vi "видео 1.vi"() -> ()   [LabVIEW 2011]
uses:
  <vilib>/userDefined/High Color/IMAQdx.ctl
  <vilib>/vision/driver/NI_Vision_Acquisition_Software.lvlib
  <vilib>/vision/NI_Vision_Development_Module.lvlib
panel:
  out "Waveform Chart":i16(graph)
  in  "Numeric":i16
  in  "milliseconds to wait":u32
  in  "Truncation Frequency %":sgl=10.0 format="%.2f"
  in  "фильтр":bool
  in  "обработка":bool
  in  "Color Box 2":u32(colorbox)
  in  "Range":cluster{"Lower value":sgl, "Upper value":sgl}={"Lower value"=128.0, "Upper value"=255.0} {"Upper value" format="%.2f"; "Lower value" format="%.2f"}
  in  "out":i32
  out "Out (dis)":string
  in  "max out":i16
  out "max Out (dis)":string
  out "Boolean":bool
  in  "vc0":i16
  in  "Регулятор":bool
  in  "PV_зазор":i32
  out "PV  зазор (мм)":string
  out "SP  зазор (мм)":string
  in  "SP_зазор":i16
  in  "stop 3":bool
  in  "stop 2":bool
  out "16bit integer":i16
  out "x*y":dbl
  out "x/y":dbl
  out "Distance деталь":sgl format="%.2f"
  out "Coordinate System деталь (duplicate)":T1 {"Measurement System"."Axis Reference" items=["Direct", "Indirect"]; "Measurement System"."Angle (deg)" format="%.2f"; "Measurement System"."Origin"."Y" format="%.2f"; "Measurement System"."Origin"."X" format="%.2f"; "Reference System"."Axis Reference" items=["Direct", "Indirect"]; "Reference System"."Angle (deg)" format="%.2f"; "Reference System"."Origin"."Y" format="%.2f"; "Reference System"."Origin"."X" format="%.2f"}
  out "Edge Coordinates деталь":cluster{"X":sgl, "Y":sgl}[](array[cluster]) {"Y" format="%.2f"; "X" format="%.2f"}
  in  "Settingsдеталь":T2={"Contrast"=40, "Filter width"=4, "Steepness"=2, "Subsampling Ratio"=5, "Show Search Area"=FALSE, "Show Search Lines"=FALSE, "Show Edges Found"=FALSE, "Show Result"=TRUE}
  in  "Coordinate System деталь":T1 {"Measurement System"."Axis Reference" items=["Direct", "Indirect"]; "Measurement System"."Angle (deg)" format="%.2f"; "Measurement System"."Origin"."Y" format="%.2f"; "Measurement System"."Origin"."X" format="%.2f"; "Reference System"."Axis Reference" items=["Direct", "Indirect"]; "Reference System"."Angle (deg)" format="%.2f"; "Reference System"."Origin"."Y" format="%.2f"; "Reference System"."Origin"."X" format="%.2f"}
  in  "Rectangle деталь":T3 {"Rotation" format="%.2f"; "Left" scale=0.0..1024.0; "Right" scale=0.0..1024.0}
  in  "Color Plane":i32(ring)=1 items=["Red", "Green", "Blue", "Hue", "Saturation", "Luminance", "Value", "Intensity"]
  out "Edge Coordinates зазор":cluster{"X":sgl, "Y":sgl}[](array[cluster]) {"Y" format="%.2f"; "X" format="%.2f"}
  out "Distance зазор":sgl format="%.2f"
  out "Coordinate System зазор (duplicate)":T1 {"Measurement System"."Axis Reference" items=["Direct", "Indirect"]; "Measurement System"."Angle (deg)" format="%.2f"; "Measurement System"."Origin"."Y" format="%.2f"; "Measurement System"."Origin"."X" format="%.2f"; "Reference System"."Axis Reference" items=["Direct", "Indirect"]; "Reference System"."Angle (deg)" format="%.2f"; "Reference System"."Origin"."Y" format="%.2f"; "Reference System"."Origin"."X" format="%.2f"}
  in  "Coordinate System зазор":T1 {"Measurement System"."Axis Reference" items=["Direct", "Indirect"]; "Measurement System"."Angle (deg)" format="%.2f"; "Measurement System"."Origin"."Y" format="%.2f"; "Measurement System"."Origin"."X" format="%.2f"; "Reference System"."Axis Reference" items=["Direct", "Indirect"]; "Reference System"."Angle (deg)" format="%.2f"; "Reference System"."Origin"."Y" format="%.2f"; "Reference System"."Origin"."X" format="%.2f"}
  in  "Settings зазор":T2={"Contrast"=40, "Filter width"=4, "Steepness"=2, "Subsampling Ratio"=5, "Show Search Area"=FALSE, "Show Search Lines"=FALSE, "Show Edges Found"=FALSE, "Show Result"=TRUE}
  in  "Rectangle зазор":T3 {"Rotation" format="%.2f"; "Left" scale=0.0..1024.0; "Right" scale=0.0..1024.0}
  in  "Color Box":u32(colorbox)
  out "Image":T4(plugin-control)
  in  "stop":bool
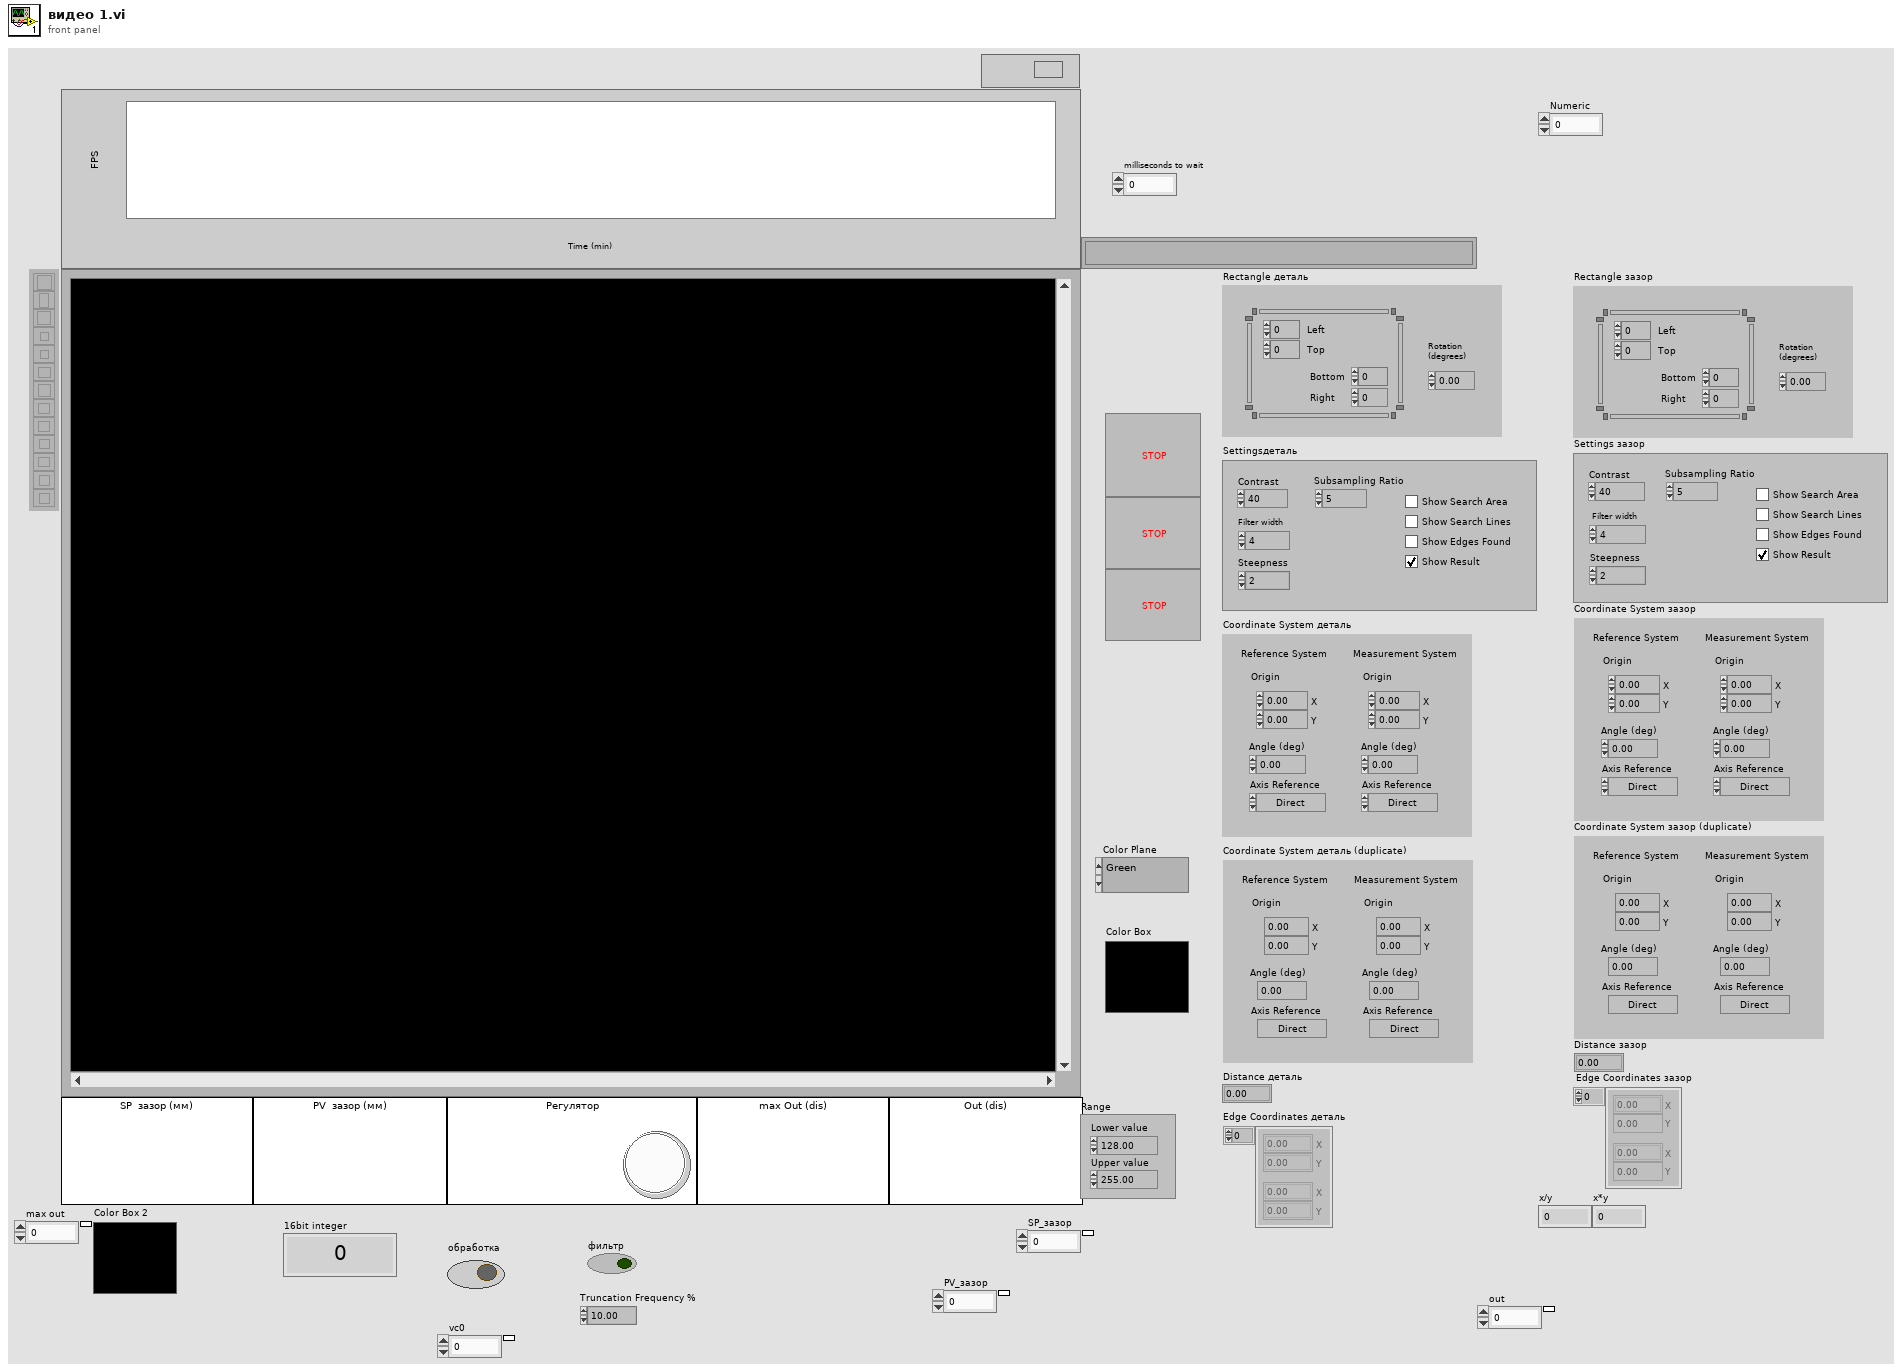
[diagram p1: front panel]
types:
  T1 = typedef "IMAQ Coordinate System" = cluster{"Reference System":cluster{"Origin":cluster{"X":sgl, "Y":sgl}, "Angle (deg)":sgl, "Axis Reference":u32}, "Measurement System":cluster{"Origin":cluster{"X":sgl, "Y":sgl}, "Angle (deg)":sgl, "Axis Reference":u32}}
  T2 = cluster{"Contrast":i32, "Filter width":i32, "Steepness":i32, "Subsampling Ratio":u32, "Show Search Area":bool, "Show Search Lines":bool, "Show Edges Found":bool, "Show Result":bool}
  T3 = typedef "IMAQ Rectangle" = cluster{"Left":i32, "Top":i32, "Right":i32, "Bottom":i32, "Rotation":dbl}
  T4 = typedef "IMAQ Image.ctl" = refnum<image>
  T5 = typedef "Image Type" = u32
  T6 = typedef "IMAQdx.ctl" = refnum<k21>
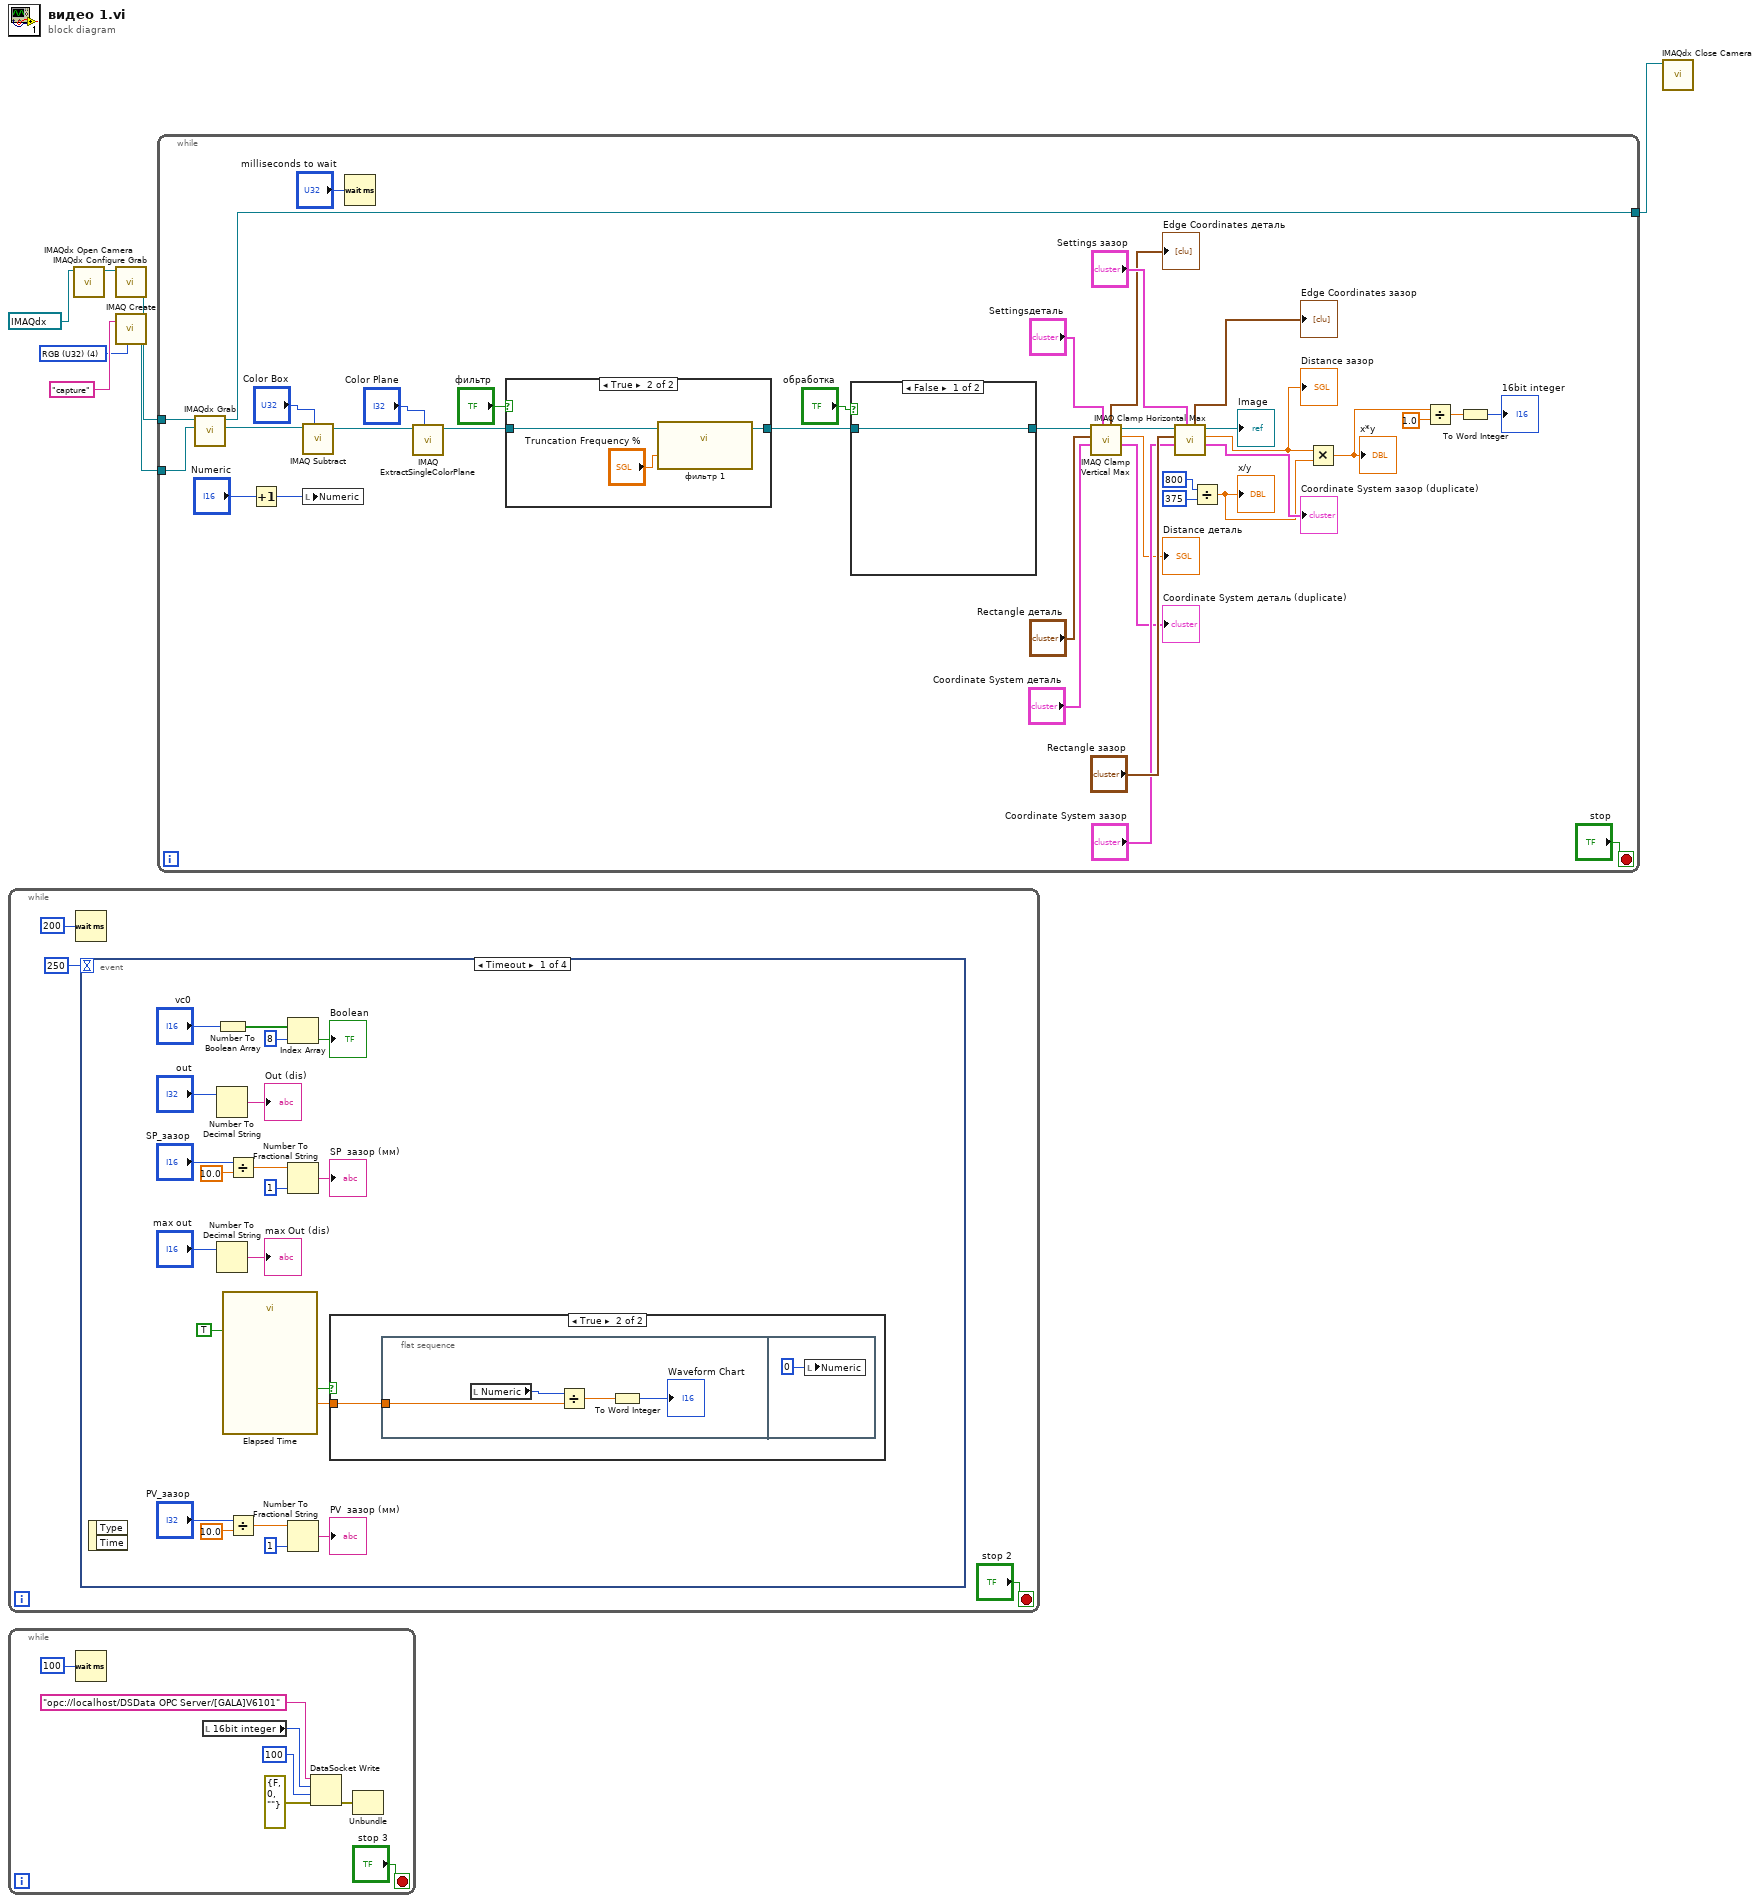
[diagram p0: block diagram]
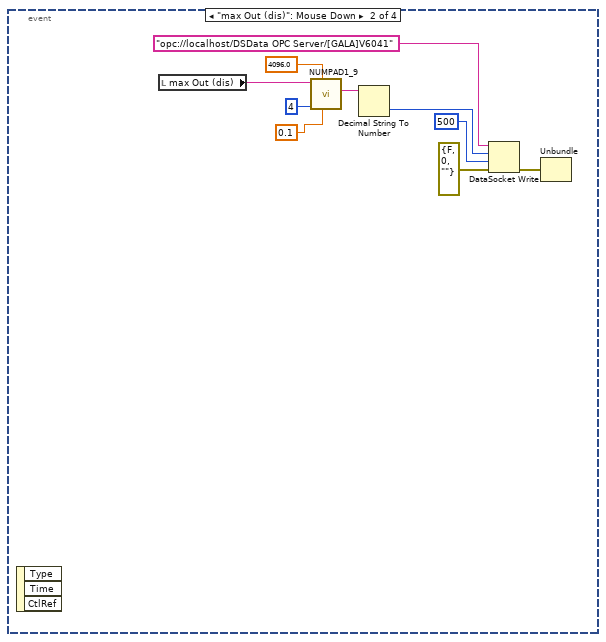
[diagram p3: hidden frame]
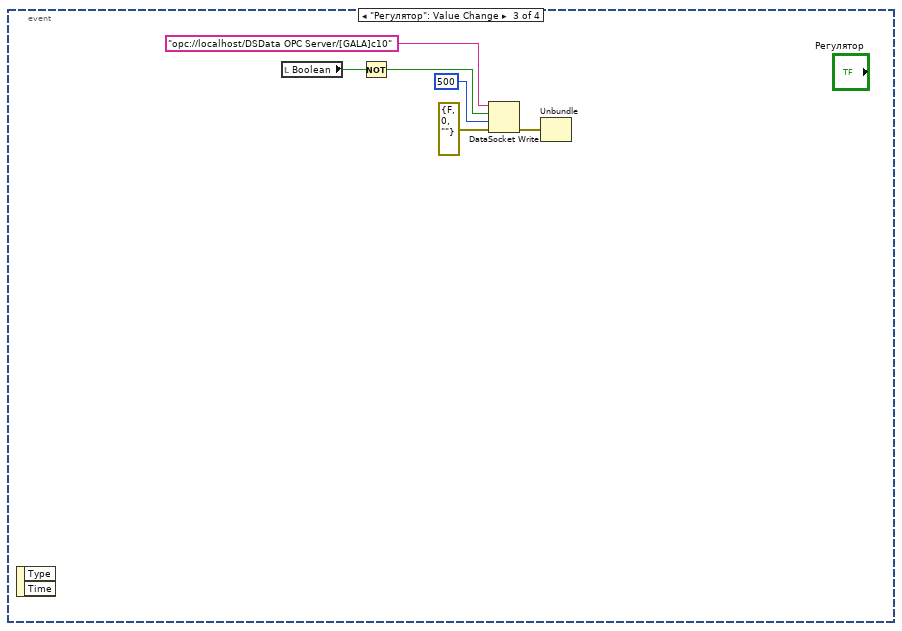
[diagram p4: hidden frame]
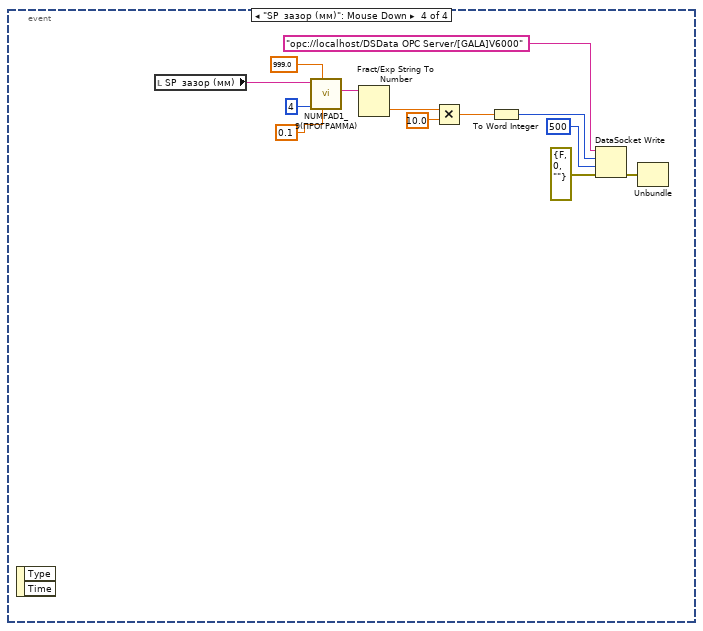
[diagram p5: hidden frame]
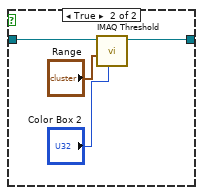
[diagram p7: hidden frame]
diagram:
  w1 = T5 4 items=["Grayscale (U8)", "Grayscale (I16)", "Grayscale (SGL)", "Complex (CSG)", "RGB (U32)", "HSL (U32)", "RGB (U64)", "Grayscale (U16)"] ("Image Type")
  n1 = while {
    stop <- "stop 2" stop-if-true
    n2 = Wait (ms)(milliseconds to wait=u32 200) -> ()  [unwired: 1 out]
    n3 = event shown="[0] Timeout" {
      selector: _ -> [_ _ _ _]
      dyn-events: _ -> [_ _ _ _]
      timeout: 250 -> [_ _ _ _]
      event Timeout {
        n4 = event-data() -> ()  [unwired: 1 in, 2 out]
        n5 = Number To Decimal String(number="out") -> (decimal integer string=→"Out (dis)":string)  [unwired: 1 in]
        n6 = Number To Decimal String(number="max out") -> (decimal integer string=→"max Out (dis)":string)  [unwired: 1 in]
        n7 = Number To Boolean Array(number="vc0") -> (Boolean array=w20:bool[])
        n8 = call "Elapsed Time"("Auto Reset"=TRUE) -> ("Elapsed Time (s)"=w12:dbl, "Time has Elapsed"=w13:bool)  [unwired: 11 in, 6 out]
        n9 = Divide(x="SP_зазор", y=10.0) -> (x/y=w29:dbl)
        n10 = Divide(x="PV_зазор", y=10.0) -> (x/y=w25:dbl)
        n11 = Index Array(array=w20, index=8) -> (element=→"Boolean":bool)
        n12 = Number To Fractional String(number=w29, precision (6)=i16 1) -> (F-format string=→"SP  зазор (мм)":string)  [unwired: 2 in]
        n13 = Number To Fractional String(number=w25, precision (6)=i16 1) -> (F-format string=→"PV  зазор (мм)":string)  [unwired: 2 in]
        n14 = case shown="True" w13 {
          tunnel: w12 -> [_ w32]
          frame False {
          }
          frame True {
            n15 = flat-sequence {
              tunnel: w32 -> [w35]
              frame #0 {
                n16 = local read "Numeric"() -> (w36:i16)
                n17 = Divide(x=w36, y=w35) -> (x/y=w34:dbl)
                n18 = To Word Integer(number=w34) -> (16bit integer=→"Waveform Chart":i16)
              }
              frame #1 {
                n19 = local write "Numeric"(i16 0 ("Numeric")) -> ()
              }
            }
          }
        }
      }
      event "max Out (dis)": Mouse Down {
        n20 = event-data() -> ()  [unwired: 1 in, 3 out]
        n21 = local read "max Out (dis)"() -> (w40:string)
        n22 = call "NUMPAD1_9.vi"("МИНИМАЛЬНОЕ ЗНАЧЕНИЕ"=0.1, "МАКСИМАЛЬНОЕ ЗНАЧЕНИЕ"=4096.0, "ДЛИННА СЛОВА"=i8 4, "ТЕКУЩЕЕ ЗНАЧЕНИЕ"=w40) -> ("НОВОЕ ЗНАЧЕНИЕ"=w39:string)  [unwired: 7 in]
        n23 = Decimal String To Number(string=w39) -> (number=w38:i32)  [unwired: 2 in, 1 out]
        n24 = DataSocket Write(8:errorcluster {"status"=FALSE, "code"=0, "source"=""} ("error in (no error)"), 9:500 ("ms timeout (0)"), 10:w38, 11:"opc://localhost/DSData OPC Server/[GALA]V6041") -> (0:w46:errorcluster)  [unwired: 2 out]
        n25 = Unbundle(w46) -> ()  [unwired: 3 out]
      }
      event "Регулятор": Value Change {
        n26 = event-data() -> ()  [unwired: 1 in, 2 out]
        n27 = local read "Boolean"() -> (w48:bool)
        n28 = Not(x=w48) -> (.not. x?=w49:bool)
        n29 = DataSocket Write(8:errorcluster {"status"=FALSE, "code"=0, "source"=""} ("error in (no error)"), 9:500 ("ms timeout (0)"), 10:w49, 11:"opc://localhost/DSData OPC Server/[GALA]c10") -> (0:w52:errorcluster)  [unwired: 2 out]
        n30 = Unbundle(w52) -> ()  [unwired: 3 out]
      }
      event "SP  зазор (мм)": Mouse Down {
        n31 = event-data() -> ()  [unwired: 1 in, 2 out]
        n32 = local read "SP  зазор (мм)"() -> (w66:string)
        n33 = call "NUMPAD1_9(ПРОГРАММА).vi"("МИНИМАЛЬНОЕ ЗНАЧЕНИЕ"=0.1, "МАКСИМАЛЬНОЕ ЗНАЧЕНИЕ"=999.0, "ДЛИННА СЛОВА"=i8 4, "ТЕКУЩЕЕ ЗНАЧЕНИЕ"=w66) -> ("НОВОЕ ЗНАЧЕНИЕ"=w63:string)  [unwired: 7 in]
        n34 = Fract/Exp String To Number(string=w63) -> (number=w62:dbl)  [unwired: 3 in, 1 out]
        n35 = Multiply(x=w62, y=10.0) -> (x*y=w60:dbl)
        n36 = To Word Integer(number=w60) -> (16bit integer=w56:i16)
        n37 = DataSocket Write(8:errorcluster {"status"=FALSE, "code"=0, "source"=""} ("error in (no error)"), 9:500 ("ms timeout (0)"), 10:w56, 11:"opc://localhost/DSData OPC Server/[GALA]V6000") -> (0:w58:errorcluster)  [unwired: 2 out]
        n38 = Unbundle(w58) -> ()  [unwired: 3 out]
      }
    }
  }
  n39 = while {
    stop <- "stop 3" stop-if-true
    n40 = Wait (ms)(milliseconds to wait=u32 100) -> ()  [unwired: 1 out]
    n41 = local read "16bit integer"() -> (w68:i16)
    n42 = DataSocket Write(8:errorcluster {"status"=FALSE, "code"=0, "source"=""} ("error in (no error)"), 9:100 ("ms timeout (0)"), 10:w68, 11:"opc://localhost/DSData OPC Server/[GALA]V6101") -> (0:w69:errorcluster)  [unwired: 2 out]
    n43 = Unbundle(w69) -> ()  [unwired: 3 out]
  }
  n44 = call <vilib>:"IMAQdx Open Camera.vi"("Session In"=T6 "cam2") -> ("Session Out"=w4:T6)  [unwired: 9 in, 1 out]
  n45 = call <vilib>:"IMAQdx Configure Grab.vi"("Session In"=w4) -> ("Session Out"=w3:T6)  [unwired: 9 in, 1 out]
  n46 = call "IMAQ Create"("Image Name"="capture", "Image Type"=w1) -> ("New Image"=w5:T4)  [unwired: 3 in, 1 out]
  n47 = while {
    tunnel: w3 -> [w109]
    tunnel: [w108] -> w7
    tunnel: w5 -> [w107]
    stop <- "stop" stop-if-true
    n48 = call <vilib>:"IMAQdx Grab.vi"("Image In"=w107, "Session In"=w109) -> ("Image Out"=w74:T4, "Session Out"=w108:T6)  [unwired: 6 in, 2 out]
    n49 = Increment(x="Numeric") -> (x+1=w75:i16)
    n50 = call "IMAQ Subtract"("Image Src A"=w74, "Constant"="Color Box") -> ("Image Dst Out"=w101:T4)  [unwired: 5 in, 1 out]
    n51 = local write "Numeric"(w75) -> ()
    n52 = Wait (ms)(milliseconds to wait="milliseconds to wait") -> ()  [unwired: 1 out]
    n53 = call "IMAQ ExtractSingleColorPlane"("Color Plane"="Color Plane", "Image Src"=w101) -> ("Image Dst Out"=w82:T4)  [unwired: 8 in, 1 out]
    n54 = case shown="True" "фильтр" {
      tunnel: w82 -> [w111 w114]
      tunnel: [w111 w113] -> w81
      frame False {
      }
      frame True {
        n55 = call "фильтр 1.vi"("Image In"=w114, "Truncation Frequency %"="Truncation Frequency %") -> ("Image Out"=w113:T4)  [unwired: 24 in, 1 out]
      }
    }
    n56 = case shown="False" "обработка" {
      tunnel: w81 -> [w115 w119]
      tunnel: [w115 w118] -> w84
      frame False {
      }
      frame True {
        n57 = call "IMAQ Threshold"("Replace Value"="Color Box 2", "Range"="Range", "Image Src"=w119) -> ("Image Dst Out"=w118:T4)  [unwired: 3 in, 5 out]
      }
    }
    n58 = call "IMAQ Clamp Vertical Max"("Settings"="Settingsдеталь", "Coordinate System"="Coordinate System деталь", "Rectangle"="Rectangle деталь", "Image"=w84) -> ("Coordinate System (duplicate)"=→"Coordinate System деталь (duplicate)":T1, "Distance"=→"Distance деталь":sgl, "Image Out"=w97:T4, "Edge Coordinates"=→"Edge Coordinates деталь":cluster{"X":sgl, "Y":sgl}[])  [unwired: 3 in, 1 out]
    n59 = call "IMAQ Clamp Horizontal Max"("Settings"="Settings зазор", "Coordinate System"="Coordinate System зазор", "Rectangle"="Rectangle зазор", "Image"=w97) -> ("Coordinate System (duplicate)"=→"Coordinate System зазор (duplicate)":T1, "Distance"=w90:sgl, "Image Out"=→"Image":T4, "Edge Coordinates"=→"Edge Coordinates зазор":cluster{"X":sgl, "Y":sgl}[])  [unwired: 3 in, 1 out]
    "Distance зазор" <- w90
    n60 = Divide(x=800, y=375) -> (x/y=w89:dbl)
    "x/y" <- w89
    n61 = Multiply(x=w90, y=w89) -> (x*y=w87:dbl)
    "x*y" <- w87
    n62 = Divide(x=w87, y=1.0) -> (x/y=w85:dbl)
    n63 = To Word Integer(number=w85) -> (16bit integer=→"16bit integer":i16)
  }
  n64 = call <vilib>:"IMAQdx Close Camera.vi"("Session In"=w7) -> ()  [unwired: 10 in, 1 out]
